vi "Find Supported Comm.vi"(8 "error in (no error)":errorcluster) -> (0 "error out":errorcluster, 2 "Supported Cameras":string[](array[string]), 3 "Camera Driver Paths":path[](array[path]))   [LabVIEW 2021]
uses:
  <vilib>/Utility/error.llb/Error Cluster From Error Code.vi
  <vilib>/ErrorRing/Error Ring.xnode
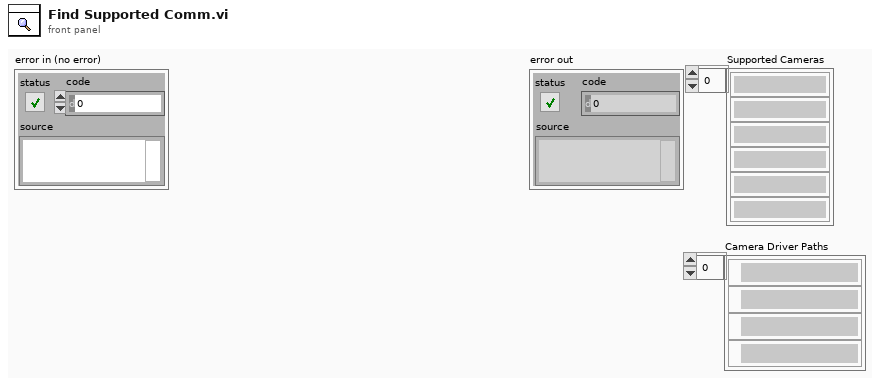
[diagram p1: front panel]
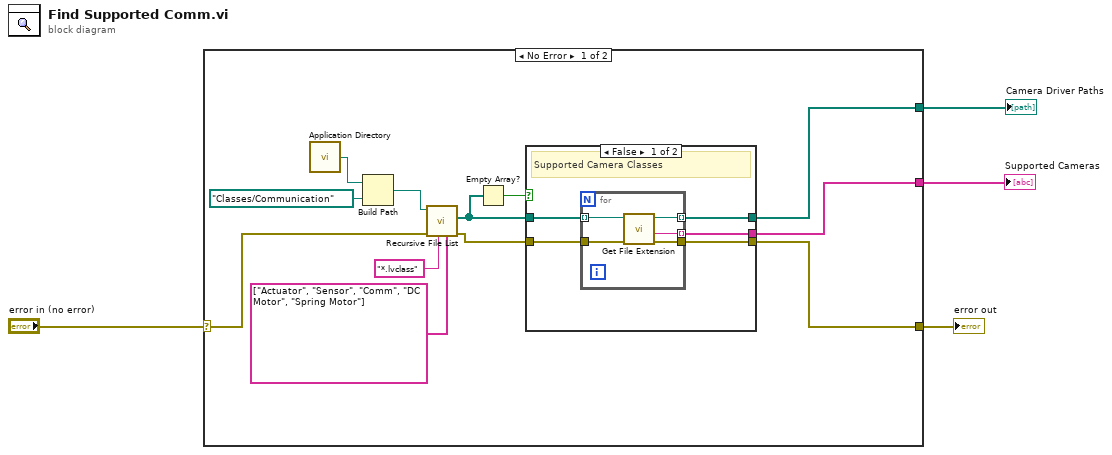
[diagram p0: block diagram]
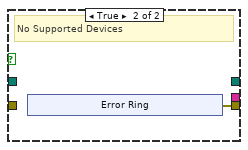
[diagram p2: hidden frame]
diagram:
  n1 = case shown="No Error" "error in (no error)" {
    selector: "error in (no error)" -> [w10 w33]
    tunnel: [w14 w33] -> w4
    tunnel: [w9 _] -> w2
    tunnel: [w8 _] -> w1
    frame No Error {
      n2 = call <vilib>:"Application Directory.vi"() -> ("Application Directory"=w7:path)
      n3 = Build Path(base path=w7, name or relative path=path "Classes/Communication") -> (appended path=w6:path)
      n4 = call <vilib>:"Recursive File List.vi"("Folders to Exclude"=string[] ["Actuator", "Sensor", "Comm", "DC Motor", "Spring Motor"], "pattern"="*.lvclass", "error in (no error)"=w10, "Folder Path"=w6) -> ("error out"=w11:errorcluster, "All Files in Dir"=w13:path[])  [unwired: 3 in, 3 out]
      n5 = Empty Array?(array=w13) -> (empty?=w12:bool)
      n6 = case shown="False" w12 {
        tunnel: [w21 w27] -> w14
        tunnel: w13 -> [w20 _]
        tunnel: w11 -> [w19 _]
        tunnel: [w18 _] -> w8
        tunnel: [w17 _] -> w9
        frame False {
          # "Supported Camera Classes"
          n7 = for {
            tunnel: [w26] -> w18 mode=indexing
            tunnel: w20 -> [w25] mode=indexing
            tunnel: [w24] -> w17 mode=indexing
            tunnel: [w23] -> w21
            tunnel: w19 -> [w22]
            n8 = call <vilib>:"Get File Extension.vi"("error in (no error)"=w22, "file"=w25) -> ("error out"=w23:errorcluster, "filename without extension"=w26:string, "dup file"=w24:path)  [unwired: 5 in, 2 out]
          }
        }
        frame True {
          # "No Supported Devices"
          n9 = xnode "Error Ring"() -> ("error out"=w27:errorcluster)
        }
      }
    }
    frame Error {
    }
  }
  "error out" <- w4
  "Camera Driver Paths" <- w2
  "Supported Cameras" <- w1
